vi "ViewTDMS.vi"   [LabVIEW 2012]
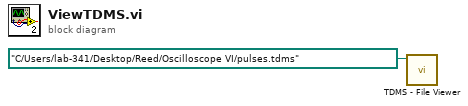
[diagram p0: block diagram]
diagram:
  n1 = call <vilib>:"TDMS - File Viewer.vi"("file path"=path "C:/Users/lab-341/Desktop/Reed/Oscilloscope VI/pulses.tdms") -> ()  [unwired: 5 in, 2 out]
